vi "Read gesture + speed - Leap.vi"() -> ()   [LabVIEW 2014]
uses:
  <vilib>/Utility/file.llb/Write To Spreadsheet File (DBL).vi
panel:
  in  "Save":bool
  out "velocità medie finali":T1(graph)
  out "velocità medie istantanee":T2(graph)
  in  "Acquire":bool
  out "Finger pinch":bool[](array[boolean])
  out "Key tap":string[](array[string])=["Undetected", "Undetected", "Undetected", "Undetected", "Undetected"]
  in  "Key Tap Thresh [degree]":sgl=55.0 caption="Key Tap Threshold [degree]"
  out "Wrist Flexion/Extension":string="Undetected"
  in  "Flex Extension Thresh [degree]":sgl=40.0
  out "Palm State":string="Undetected"
  in  "Stop":bool
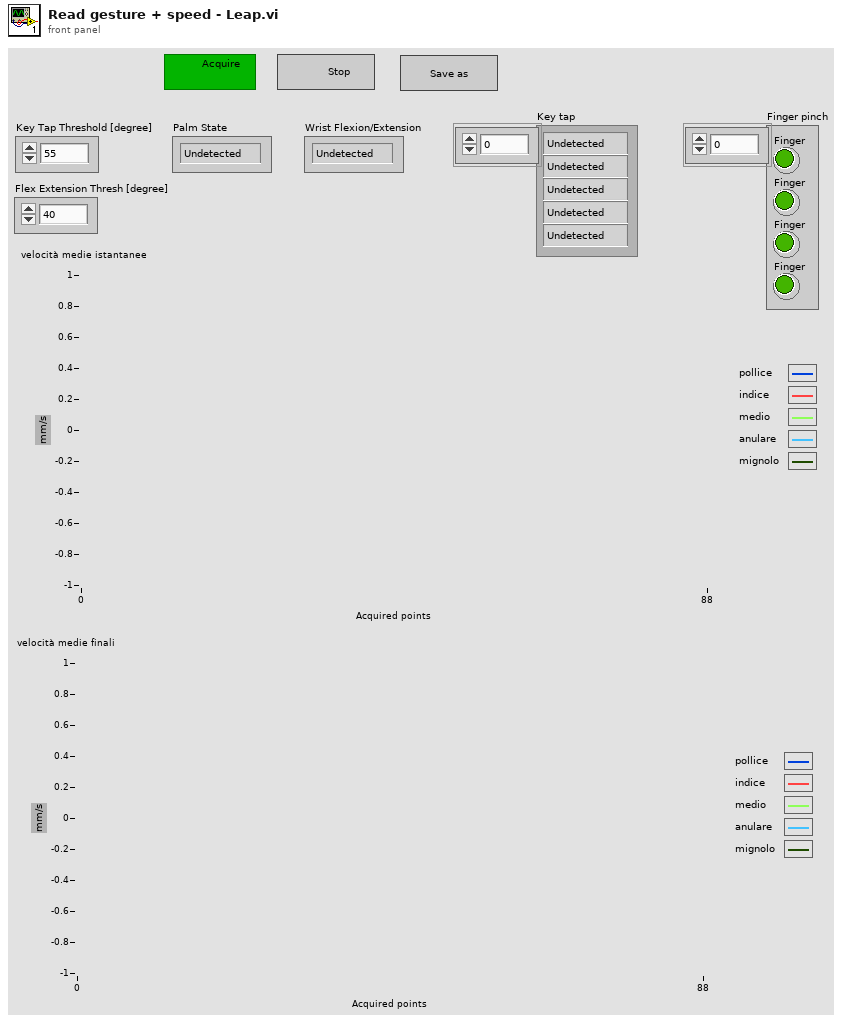
[diagram p1: front panel]
types:
  T1 = cluster{"sqrt(x)":sgl, "sqrt(x)":sgl, "sqrt(x)":sgl, "sqrt(x)":sgl, "sqrt(x)":sgl}
  T2 = cluster{"mean":dbl, "mean":dbl, "mean":dbl, "mean":dbl, "mean":dbl}
  T3 = typedef "Leap Handle.ctl" = cluster{"LeapCSharp":refnum<k24>}
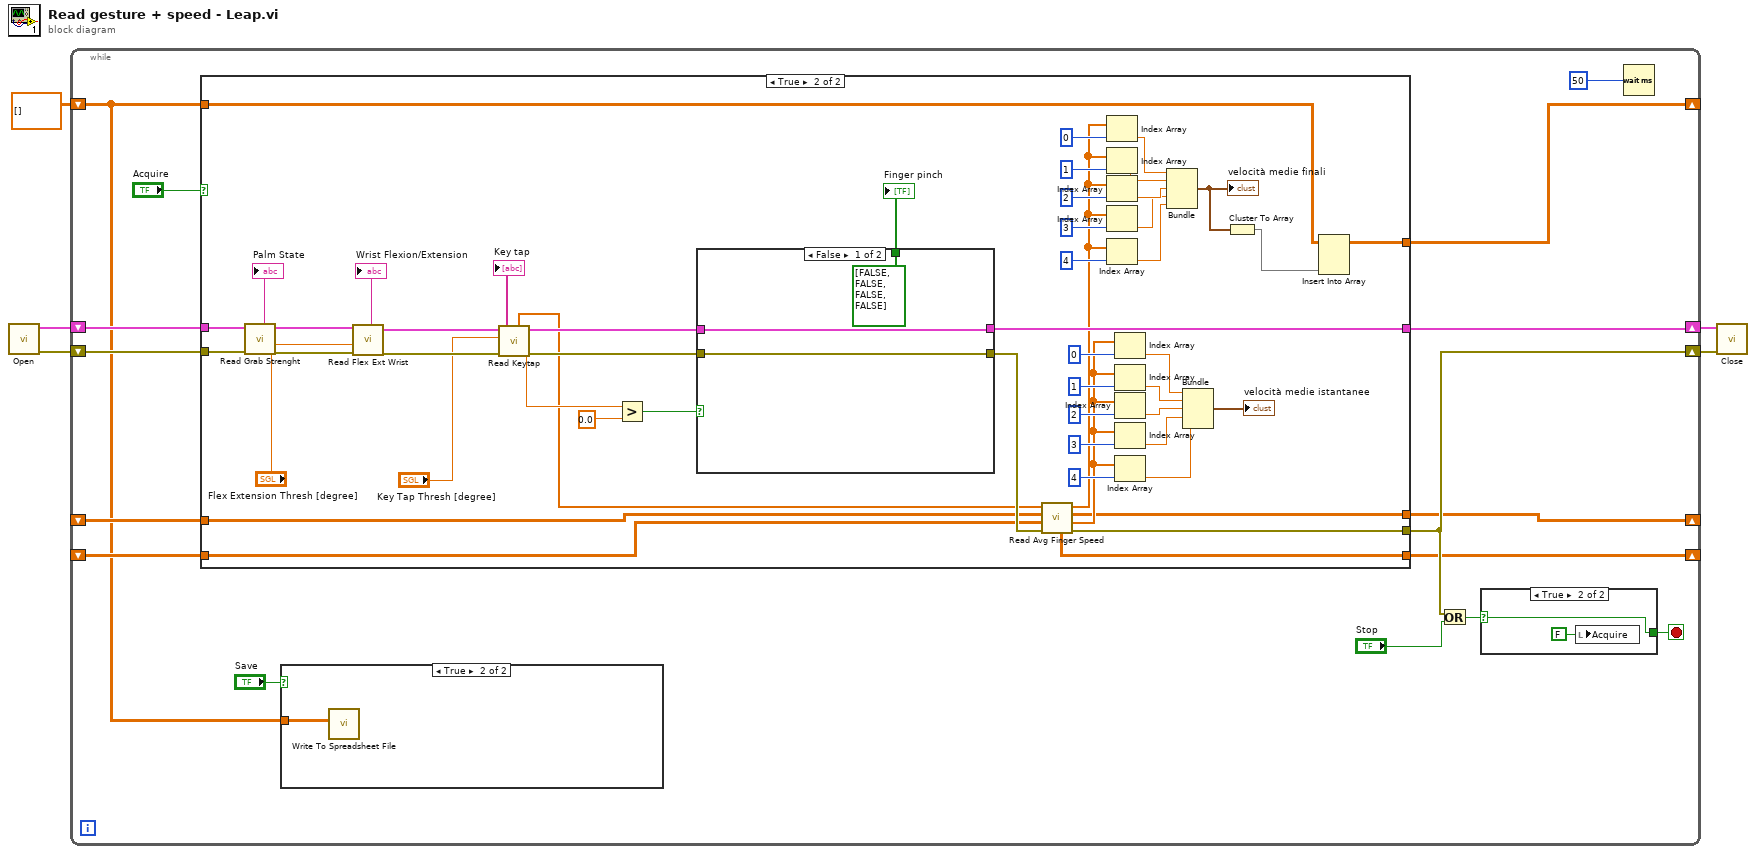
[diagram p0: block diagram]
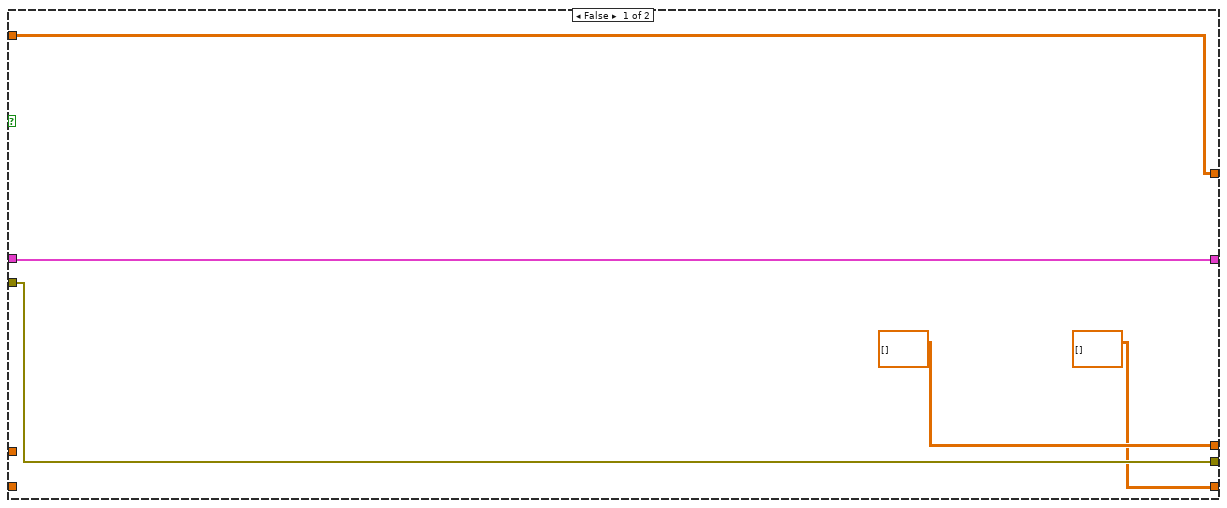
[diagram p4: hidden frame]
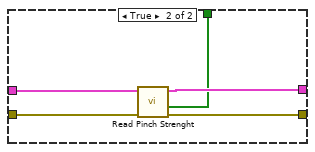
[diagram p5: hidden frame]
diagram:
  n1 = call "Open.vi"() -> ("Error Out"=w4:errorcluster, "Leap Handle"=w5:T3)  [unwired: 10 in]
  n2 = while {
    shift-right: [w17] -> w3
    shift-left: w5 -> [w16]
    shift-right: [w18] -> w2
    shift-left: w4 -> [w19]
    shift-right: [w12] -> _
    shift-left: _ -> [w11]
    shift-right: [w10] -> _
    shift-left: _ -> [w9]
    shift-right: [w8] -> _
    shift-left: sgl[][] [] -> [w7]
    stop <- w13 stop-if-true
    n3 = case shown="True" "Acquire" {
      tunnel: w19 -> [w29 w82]
      tunnel: [w29 w40] -> w18
      tunnel: [w30 w69] -> w17
      tunnel: w16 -> [w30 w68]
      tunnel: [sgl[][] [] ("Array OUT") w42] -> w12
      tunnel: w11 -> [_ w44]
      tunnel: [sgl[][] [] ("Array vel medie") w39] -> w10
      tunnel: w9 -> [_ w38]
      tunnel: [w26 w32] -> w8
      tunnel: w7 -> [w26 w31]
      frame False {
      }
      frame True {
        n4 = call "Read Grab Strenght.vi"("Error In"=w82, "Leap Handle In"=w68) -> ("Error Out"=w79:errorcluster, "Leap Handle Out"=w80:T3, "Palm State"=→"Palm State":string)  [unwired: 5 in, 2 out]
        n5 = call "Read Flex Ext Wrist.vi"("Error In"=w79, "Flex Extension threshold"="Flex Extension Thresh [degree]", "Leap Handle In"=w80) -> ("Error Out"=w76:errorcluster, "Wrist Flextion/Extension"=→"Wrist Flexion/Extension":string, "Leap Handle Out"=w77:T3)  [unwired: 4 in]
        n6 = call "Read Keytap.vi"("Error In"=w76, "Key Tap Thresh"="Key Tap Thresh [degree]", "Leap Handle In"=w77) -> ("Error Out"=w73:errorcluster, "PinchStrength"=w71:sgl, "Key tap"=→"Key tap":string[], "Leap Handle Out"=w74:T3, "Tip Velocity Module"=w35:dbl[])  [unwired: 3 in]
        n7 = Greater?(x=w71, y=0.0) -> (0:w72:bool)
        n8 = case shown="False" w72 {
          tunnel: w74 -> [w85 w88]
          tunnel: w73 -> [w84 w90]
          tunnel: [w84 w89] -> w45
          tunnel: [w85 w87] -> w69
          tunnel: [bool[] [FALSE, FALSE, FALSE, FALSE] ("Finger pinch") w86] -> w70
          frame False {
          }
          frame True {
            n9 = call "Read Pinch Strenght.vi"("Error In"=w90, "Leap Handle In"=w88) -> ("Error Out"=w89:errorcluster, "Finger pinch"=w86:bool[], "Leap Handle Out"=w87:T3)  [unwired: 6 in, 1 out]
          }
        }
        "Finger pinch" <- w70
        n10 = call "Read Avg Finger Speed.vi"("Tip Velocity Module"=w35, "Array v istantanee  IN"=w44, "Array vel medie IN"=w38, "Error In"=w45) -> ("Array vel medie OUT"=w39:sgl[][], "Velocità medie finali"=w41:sgl[], "Array v istantanee OUT"=w42:sgl[][], "velocità medie istantanee out"=w43:dbl[], "Error Out"=w40:errorcluster)  [unwired: 1 in]
        n11 = Index Array(array=w41, index=0) -> (element=w50:sgl)
        n12 = Index Array(array=w41, index=1) -> (element=w49:sgl)
        n13 = Index Array(array=w41, index=2) -> (element=w48:sgl)
        n14 = Index Array(array=w41, index=3) -> (element=w47:sgl)
        n15 = Index Array(array=w41, index=4) -> (element=w46:sgl)
        n16 = Index Array(array=w43, index=0) -> (element=w61:dbl)
        n17 = Index Array(array=w43, index=1) -> (element=w60:dbl)
        n18 = Index Array(array=w43, index=2) -> (element=w59:dbl)
        n19 = Index Array(array=w43, index=3) -> (element=w58:dbl)
        n20 = Index Array(array=w43, index=4) -> (element=w57:dbl)
        n21 = Bundle("sqrt(x)"=w50, "sqrt(x)"=w49, "sqrt(x)"=w48, "sqrt(x)"=w47, "sqrt(x)"=w46) -> (w34:T1)  [unwired: 1 in]
        "velocità medie finali" <- w34
        n22 = Bundle("mean"=w61, "mean"=w60, "mean"=w59, "mean"=w58, "mean"=w57) -> (→"velocità medie istantanee":T2)  [unwired: 1 in]
        n23 = Cluster To Array(cluster=w34) -> (array=w33:sgl[])
        n24 = Insert Into Array(array=w31, new element=w33) -> (w32:sgl[][])  [unwired: 2 in]
      }
    }
    n25 = case shown="True" "Save" {
      tunnel: w7 -> [_ w22]
      frame False {
      }
      frame True {
        n26 = call-poly <vilib>:"Write To Spreadsheet File.vi"("2D data"=w22) -> ()  [unwired: 7 in, 1 out]
      }
    }
    n27 = Or(x=w18, y="Stop") -> (x .or. y?=w14:bool)
    n28 = case shown="True" w14 {
      selector: w14 -> [w23 w24]
      tunnel: [w23 w24] -> w13
      frame False {
      }
      frame True {
        n29 = local write "Acquire"(FALSE ("Acquire")) -> ()
      }
    }
    n30 = Wait (ms)(milliseconds to wait=u32 50) -> ()  [unwired: 1 out]
  }
  n31 = call "Close.vi"("Error In"=w2, "Leap Handle"=w3) -> ()  [unwired: 9 in, 1 out]
